vi "Configure Arbitrary Waveform.vi"(4 "Frequency (1000 Hz)":dbl=1000.0, 6 "DC Offset (0 V)":dbl, 7 "Arbitrary Waveform Name (0: USER1)":u16(ring) items=["USER1", "USER2", "USER3", "USER4"], 8 "error in (no error)":errorcluster, 9 "Gain (1 V)":dbl=1.0, 10 "Channel (0: Channel 1)":u16(ring) items=["Channel 1", "Channel 2"], 11 "VISA resource name":refnum<visa-resource-name>) -> (0 "error out":errorcluster, 3 "VISA resource name out":refnum<visa-resource-name>)   [LabVIEW 2019, in "Tektronix AFG 3000 Series.lvlib"]
doc: "Configures the function generator settings that affect arbitrary waveform generation."
uses:
  <userlib>/Tektronix AFG 3000 Series/Tektronix AFG 3000 Series.lvlib
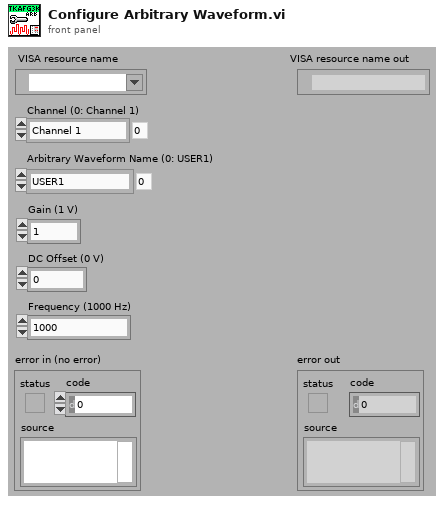
[diagram p1: front panel]
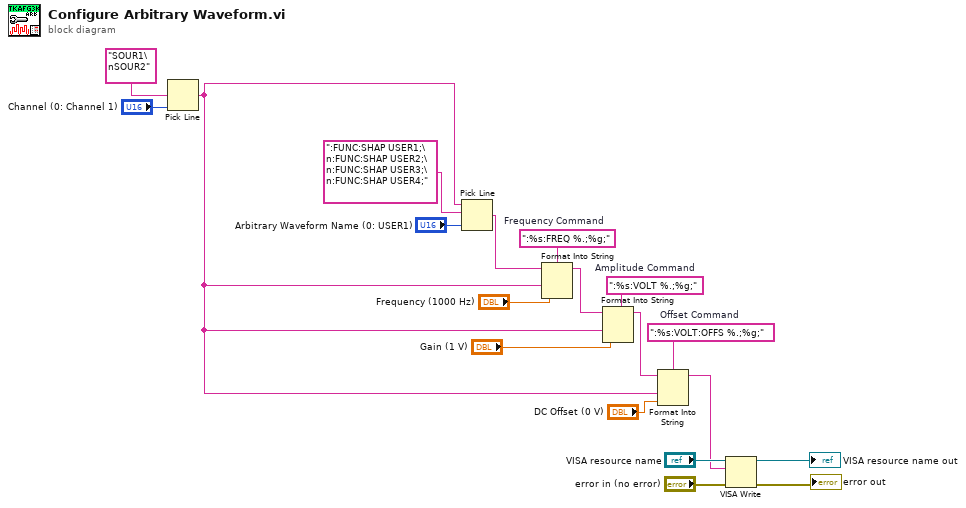
[diagram p0: block diagram]
diagram:
  w7 = ":%s:VOLT:OFFS %.;%g;"  # Offset Command
  w8 = ":%s:VOLT %.;%g;"  # Amplitude Command
  w9 = ":%s:FREQ %.;%g;"  # Frequency Command
  n1 = Pick Line(multi-line string="SOUR1\nSOUR2" ("string (\"\")"), line index="Channel (0: Channel 1)") -> (output string=w3:string)  [unwired: 1 in]
  n2 = Pick Line(string ("")=w3, multi-line string=":FUNC:SHAP USER1;\n:FUNC:SHAP USER2;\n:FUNC:SHAP USER3;\n:FUNC:SHAP USER4;" ("string (\"\")"), line index="Arbitrary Waveform Name (0: USER1)") -> (output string=w10:string)
  n3 = Format Into String(format string=w9, initial string=w10, w3, "Frequency (1000 Hz)") -> (resulting string=w14:string)  [unwired: 1 in, 1 out]
  n4 = Format Into String(format string=w8, initial string=w14, w3, "Gain (1 V)") -> (resulting string=w13:string)  [unwired: 1 in, 1 out]
  n5 = Format Into String(format string=w7, initial string=w13, w3, "DC Offset (0 V)") -> (resulting string=w17:string)  [unwired: 1 in, 1 out]
  n6 = VISA Write(VISA resource name="VISA resource name", write buffer=w17, error in (no error)="error in (no error)") -> (VISA resource name out=→"VISA resource name out":refnum<visa-resource-name>, error out=→"error out":errorcluster)  [unwired: 1 out]
